vi "main.vi"() -> ()   [LabVIEW 2016]
uses:
  <vilib>/Utility/config.llb/Read Key (String).vi
  <vilib>/Utility/config.llb/Write Key (String).vi
  <vilib>/Utility/config.llb/NI_LVConfig.lvlib
  <vilib>/ptbypt/NI_PtbyPt.lvlib
panel:
  in  "Password":string="783523103"
  in  "日数据table表":string="t_sjzx_wryzxjc_fs_rsj"
  in  "connection information":string="mysql"
  out "计数":i32
  out "数值":i32
  out "time":string
  out "error out":errorcluster
  in  "修改数据发送起始时间":bool
  in  "因子编码表":bool
  in  "QYMC-企业名称":string="安徽晨蓝环保科技有限公司（凤台经济开发区污水处理厂）"
  in  "QYBH-企业编号":string="340100000133"
  in  "PKMC-排口名称":string="污水排口"
  in  "PKBH-排口编号":string="340400000010WaterOutput2"
  in  "XH-序号":string="34040000001020012018103012"
  in  "小时数据table表":string="t_sjzx_wryzxjc_fs_xssj"
  out "参数table":string
  out "数据时间":string[](array[string])
  in  "等待时间（毫秒）":u32=30000
  in  "参数数值":T1={"CODMn"=TRUE, "CODCr"=TRUE, "DO"=TRUE, "铜"=TRUE, "PH"=TRUE, "氨氮"=TRUE, "比电导率"=TRUE, "水温"=TRUE, "COD"=TRUE, "浊度"=TRUE, "总氮"=TRUE, "总磷"=TRUE, "叶绿素a"=TRUE, "藻密度"=TRUE, "水位"=TRUE, "流速"=TRUE, "瞬时流量"=TRUE, "累积流量"=TRUE, "亚硝氮"=TRUE, "硫化物"=TRUE, "ORP"=TRUE, "铅"=TRUE, "镉"=TRUE, "锌"=TRUE, "镍"=TRUE, "锰"=TRUE, "汞"=TRUE, "气温"=TRUE, "气压"=TRUE, "风速"=TRUE, "风向"=TRUE} caption="参数种类"
  # "定时分参数循环读取database数据------------->多条数据分条转换循环存储到mysql数据库中------->成功则更新搜索时间戳、失败不更新"
  # "示例：34040000001020012018103012"
  # "示例：340400000010WaterOutput2"
  # "示例：污水排口"
  # "示例：340100000133"
  # "示例：安徽晨蓝环保科技有限公司（凤台经济开发区污水处理厂）"
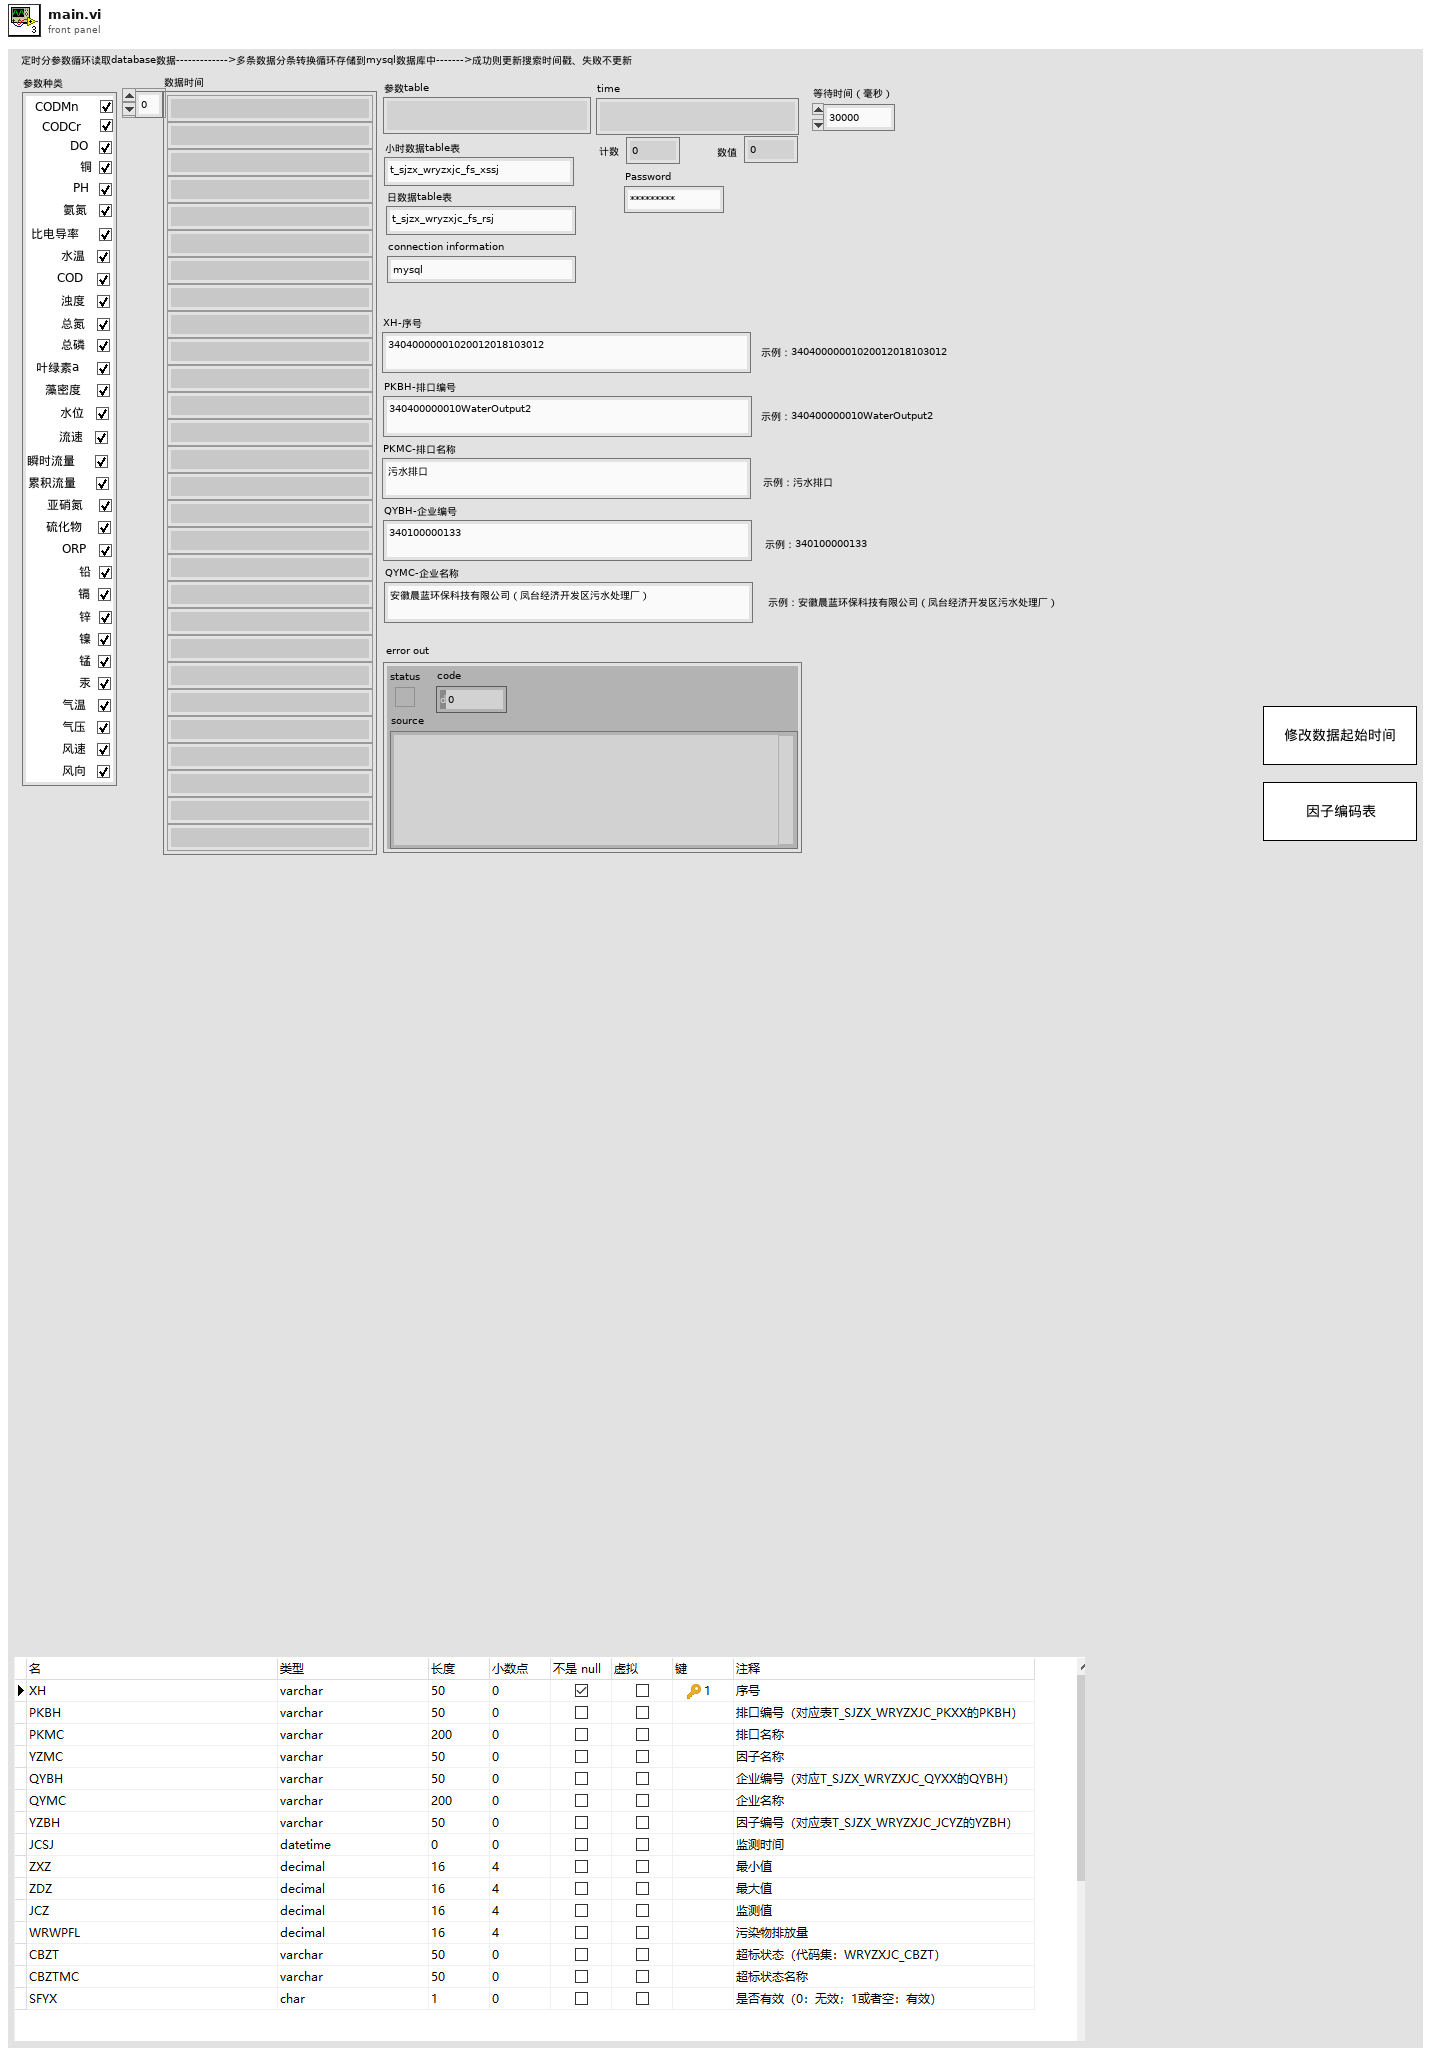
[diagram p1: front panel]
types:
  T1 = cluster{"CODMn":bool, "CODCr":bool, "DO":bool, "铜":bool, "PH":bool, "氨氮":bool, "比电导率":bool, "水温":bool, "COD":bool, "浊度":bool, "总氮":bool, "总磷":bool, "叶绿素a":bool, "藻密度":bool, "水位":bool, "流速":bool, "瞬时流量":bool, "累积流量":bool, "亚硝氮":bool, "硫化物":bool, "ORP":bool, "铅":bool, "镉":bool, "锌":bool, "镍":bool, "锰":bool, "汞":bool, "气温":bool, "气压":bool, "风速":bool, "风向":bool}
  T2 = typedef "NI_LVConfig.lvlib/Config Data RefNum.ctl" = refnum<k1>
  T3 = cluster{"[0]":string, "[1]":string, "[2]":string, "[3]":string, "[4]":string, "[5]":string, "[6]":string, "[7]":string, "[8]":string, "[9]":string, "[10]":string, "[11]":string, "[12]":string, "[13]":string, "[14]":string, "[15]":string, "[16]":string, "[17]":string, "[18]":string, "[19]":string, "[20]":string, "[21]":string, "[22]":string, "[23]":string, "[24]":string, "[25]":string, "[26]":string, "[27]":string, "[28]":string, "[29]":string, "[30]":string}
  T4 = typedef "LVDateTimeRec.ctl" = cluster{"秒数的小数部分":dbl, "秒":i32, "分":i32, "时":i32, "日":i32, "月":i32, "年":i32, "天数（周）":i32, "天数（年）":i32, "DST":i32}
  T5 = cluster{"CODMn":string, "CODCr":string, "DO":string, "铜":string, "PH":string, "氨氮":string, "比电导率":string, "水温":string, "COD":string, "浊度":string, "总氮":string, "总磷":string, "叶绿素a":string, "藻密度":string, "水位":string, "流速":string, "瞬时流量":string, "累积流量":string, "亚硝酸盐":string, "硫化物":string, "ORP":string, "铅":string, "镉":string, "锌":string, "镍":string, "锰":string, "汞":string, "气温":string, "气压":string, "风速":string, "风向":string}
  T6 = cluster{"XH":string, "PKBH":string, "PKMC":string, "YZBH":string, "YZMC":string, "QYBH":string, "QYMC":string, "JCSJ":timestamp, "JCZ":dbl}
  T7 = cluster{"time1":string, "time2":string, "time3":string, "time4":string, "time5":string, "time6":string, "time7":string, "time8":string, "time9":string, "time10":string, "time11":string, "time12":string, "time13":string, "time14":string, "time15":string, "time16":string, "time17":string, "time18":string, "time19":string, "time20":string, "time21":string, "time22":string, "time23":string, "time24":string, "time25":string, "time26":string, "time27":string, "time28":string, "time29":string, "time30":string, "time31":string}
  T8 = cluster{"XH":string, "PKBH":string, "PKMC":string, "YZMC":string, "QYBH":string, "QYMC":string, "YZBH":string, "JCSJ":timestamp, "JCZ":dbl}
  T9 = cluster{"配置表格[0]":string, "配置表格[1]":string, "配置表格[2]":string, "配置表格[3]":string, "配置表格[4]":string, "配置表格[5]":string, "配置表格[6]":string, "配置表格[7]":string, "配置表格[8]":string, "配置表格[9]":string, "配置表格[10]":string, "配置表格[11]":string, "配置表格[12]":string, "配置表格[13]":string, "配置表格[14]":string, "配置表格[15]":string, "配置表格[16]":string, "配置表格[17]":string, "配置表格[18]":string, "配置表格[19]":string, "配置表格[20]":string, "配置表格[21]":string, "配置表格[22]":string, "配置表格[23]":string, "配置表格[24]":string, "配置表格[25]":string, "配置表格[26]":string, "配置表格[27]":string, "配置表格[28]":string, "配置表格[29]":string, "配置表格[30]":string}
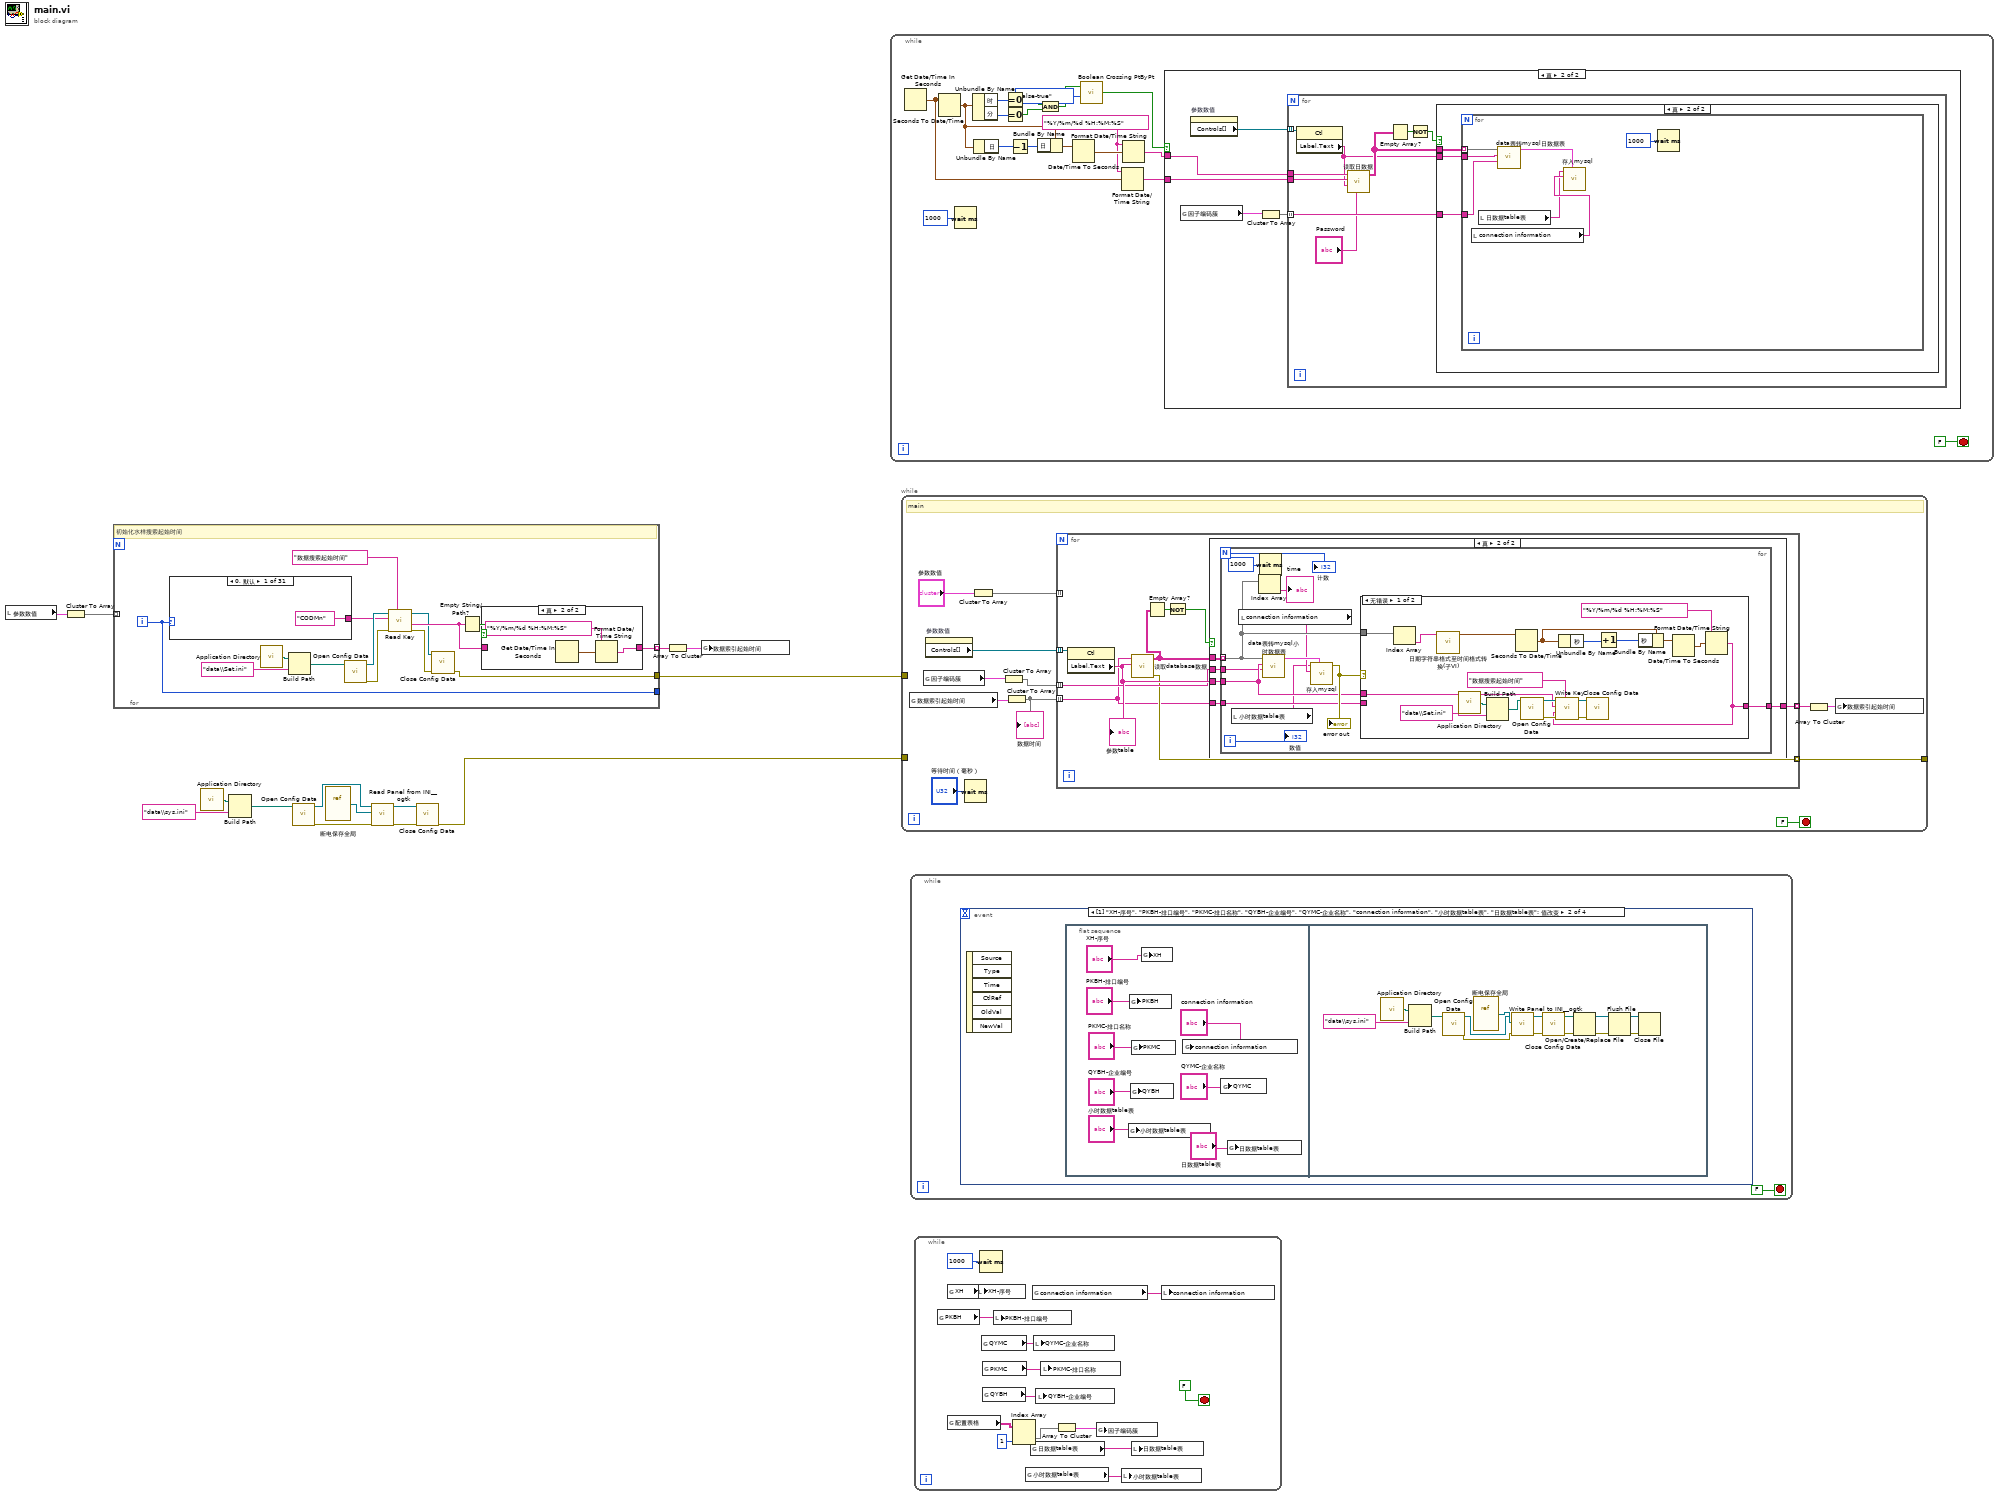
[diagram p0: block diagram]
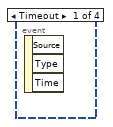
[diagram p4: hidden frame]
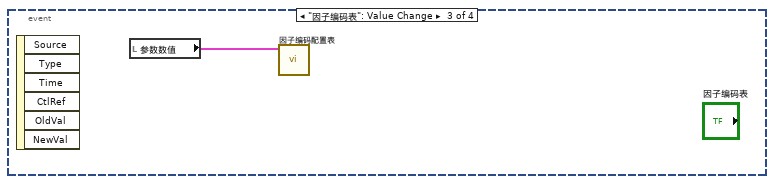
[diagram p5: hidden frame]
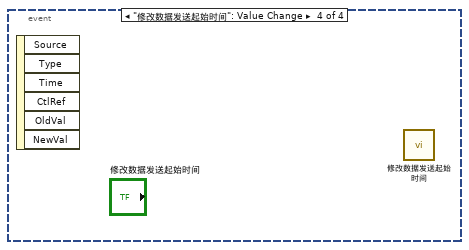
[diagram p6: hidden frame]
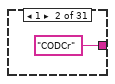
[diagram p8: hidden frame]
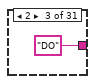
[diagram p9: hidden frame]
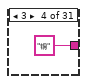
[diagram p10: hidden frame]
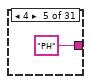
[diagram p11: hidden frame]
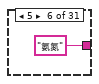
[diagram p12: hidden frame]
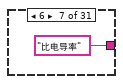
[diagram p13: hidden frame]
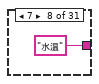
[diagram p14: hidden frame]
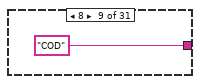
[diagram p15: hidden frame]
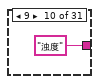
[diagram p16: hidden frame]
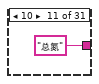
[diagram p17: hidden frame]
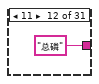
[diagram p18: hidden frame]
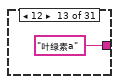
[diagram p19: hidden frame]
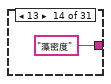
[diagram p20: hidden frame]
diagram:
  n1 = local read "参数数值"() -> (w14:T1)
  n2 = Cluster To Array(cluster=w14) -> (array=w13:bool[])
  n3 = for {
    tunnel: [w19] -> _
    tunnel: [w16] -> w12 mode=indexing
    tunnel: [w15] -> w11
    tunnel: w13 -> [_] mode=indexing
    i -> [w19]
    # "初始化水样搜索起始时间"
    n4 = case shown="0, 默认" w19 {
      tunnel: ["CODMn" "CODCr" "DO" "铜" "PH" "氨氮" "比电导率" "水温" "COD" "浊度" "总氮" "总磷" "叶绿素a" "藻密度" "水位" "流速" "瞬时流量" "累积流量" "亚硝氮" "硫化物" "ORP" "铅" "镉" "锌" "镍" "锰" "汞" "气温" "气压" "风速" "风向"] -> w22
      frame 0, Default {
      }
      frame 1 {
      }
      frame 2 {
      }
      frame 3 {
      }
      frame 4 {
      }
      frame 5 {
      }
      frame 6 {
      }
      frame 7 {
      }
      frame 8 {
      }
      frame 9 {
      }
      frame 10 {
      }
      frame 11 {
      }
      frame 12 {
      }
      frame 13 {
      }
      frame 14 {
      }
      frame 15 {
      }
      frame 16 {
      }
      frame 17 {
      }
      frame 18 {
      }
      frame 19 {
      }
      frame 20 {
      }
      frame 21 {
      }
      frame 22 {
      }
      frame 23 {
      }
      frame 24 {
      }
      frame 25 {
      }
      frame 26 {
      }
      frame 27 {
      }
      frame 28 {
      }
      frame 29 {
      }
      frame 30 {
      }
    }
    n5 = call <vilib>:"Application Directory.vi"() -> ("Application Directory"=w28:path)
    n6 = Build Path(base path=w28, name or relative path="data\\Set.ini" ("名称或相对路径")) -> (appended path=w26:path)
    n7 = call <vilib>:"Open Config Data.vi"("configuration file path"=w26) -> ("error out"=w24:errorcluster, "refnum"=w25:T2)  [unwired: 8 in, 1 out]
    n8 = call-poly <vilib>:"Read Key.vi"("section"="数据搜索起始时间", "error in (no error)"=w24, "key"=w22, "refnum"=w25) -> ("error out"=w17:errorcluster, "value"=w20:string, "refnum out"=w18:T2)  [unwired: 4 in, 1 out]
    n9 = call <vilib>:"Close Config Data.vi"("error in (no error)"=w17, "refnum"=w18) -> ("error out"=w15:errorcluster)  [unwired: 8 in, 1 out]
    n10 = Empty String/Path?(string/path=w20) -> (empty?=w21:bool)
    n11 = case shown="真" w21 {
      tunnel: [w29 w30] -> w16
      tunnel: w20 -> [w29 _]
      frame False {
      }
      frame True {
        n12 = Get Date/Time In Seconds() -> (seconds since 1Jan1904=w32:timestamp)
        n13 = Format Date/Time String(time format string (%c)="%Y/%m/%d %H:%M:%S" ("时间格式字符串(%c)"), seconds (now)=w32) -> (date/time string=w30:string)  [unwired: 1 in]
      }
    }
  }
  n14 = call <vilib>:"Application Directory.vi"() -> ("Application Directory"=w5:path)
  n15 = Build Path(base path=w5, name or relative path="data\\sys.ini" ("名称或相对路径")) -> (appended path=w3:path)
  n16 = call <vilib>:"Open Config Data.vi"("configuration file path"=w3) -> ("error out"=w9:errorcluster, "refnum"=w8:T2)  [unwired: 8 in, 1 out]
  n17 = vi-ref "断电保存全局.vi"() -> (w7:refnum<vi>)
  n18 = call <userlib>:"Read Panel from INI__ogtk.vi"("error in (no error)"=w9, "VI ref"=w7, "refnum"=w8) -> ("error out"=w2:errorcluster, "refnum out"=w6:T2)  [unwired: 7 in]
  n19 = call <vilib>:"Close Config Data.vi"("error in (no error)"=w2, "refnum"=w6) -> ("error out"=w1:errorcluster)  [unwired: 8 in, 1 out]
  n20 = Array To Cluster(array=w12) -> (cluster=w10:T3)
  n21 = global write "内部全局.vi" "数据索引起始时间"(w10) -> ()
  n22 = while {
    stop <- FALSE stop-if-true
    w70 = "%Y/%m/%d %H:%M:%S" ("时间格式字符串(%c)")
    n23 = Get Date/Time In Seconds() -> (seconds since 1Jan1904=w69:timestamp)
    n24 = Seconds To Date/Time(time stamp (now)=w69) -> (date time rec=w76:T4)  [unwired: 1 in]
    n25 = Wait (ms)(milliseconds to wait=u32 1000 ("等待时间（毫秒）")) -> ()  [unwired: 1 out]
    n26 = Unbundle By Name(w76) -> ("时"=w79:i32, "分"=w78:i32)
    n27 = Unbundle By Name(w76) -> ("日"=w75:i32)
    n28 = Equal To 0?(x=w79) -> (x = 0?=w72:bool)
    n29 = Equal To 0?(x=w78) -> (x = 0?=w73:bool)
    n30 = Decrement(x=w75) -> (x-1=w74:i32)
    n31 = Bundle By Name(cluster=w76, "日"=w74) -> (w77:T4)
    n32 = And(x=w72, y=w73) -> (x .and. y?=w66:bool)
    n33 = Date/Time To Seconds(2:w77) -> (0:w71:timestamp)  [unwired: 1 in]
    n34 = call <vilib>:"Boolean Crossing PtByPt.vi"("direction"=enum16{"either", "false-true", "true-false"}."false-true", "input"=w66) -> ("crossing"=w64:bool)  [unwired: 1 in]
    n35 = Format Date/Time String(time format string (%c)=w70, seconds (now)=w69) -> (date/time string=w67:string)  [unwired: 1 in]
    n36 = Format Date/Time String(time format string (%c)=w70, seconds (now)=w71) -> (date/time string=w68:string)  [unwired: 1 in]
    n37 = case shown="真" w64 {
      tunnel: w68 -> [_ w86]
      tunnel: w67 -> [_ w85]
      frame False {
      }
      frame True {
        n38 = global read "断电保存全局.vi" "因子编码簇"() -> (w83:T5)
        n39 = property on="参数数值" class="Clust (严格)"() -> ("Controls[]"=w84:refnum<vi>[])  [unwired: 2 in, 2 out]
        n40 = Cluster To Array(cluster=w83) -> (array=w82:string[])
        n41 = for {
          tunnel: w86 -> [w95]
          tunnel: w85 -> [w94]
          tunnel: w84 -> [w93] mode=indexing
          tunnel: w82 -> [w88] mode=indexing
          n42 = property class="Ctl"(reference=w93) -> ("Label.Text"=w89:string)  [unwired: 1 in, 2 out]
          n43 = call "读取日数据.vi"("Password"="Password", "table输入"=w89, "结束时间"=w94, "起始时间"=w95) -> ("data"=w90:string[][])  [unwired: 6 in, 1 out]
          n44 = Empty Array?(array=w90) -> (empty?=w92:bool)
          n45 = Not(x=w92) -> (.not. x?=w91:bool)
          n46 = case shown="真" w91 {
            tunnel: w90 -> [_ w98]
            tunnel: w89 -> [_ w97]
            tunnel: w88 -> [_ w96]
            frame False {
            }
            frame True {
              n47 = for {
                tunnel: w98 -> [w105] mode=indexing
                tunnel: w97 -> [w104]
                tunnel: w96 -> [w103]
                n48 = local read "connection information"() -> (w101:string)
                n49 = local read "日数据table表"() -> (w99:string)
                n50 = call "data表转mysql日数据表.vi"("YZBH"=w103, "YZMC"=w104, "data"=w105) -> ("mysqldata簇"=w102:T6)  [unwired: 8 in]
                n51 = call "存入mysql.vi"("mysqldata簇"=w102, "connection information"=w101, "table"=w99) -> ()  [unwired: 8 in, 1 out]
                n52 = Wait (ms)(milliseconds to wait=u32 1000 ("等待时间（毫秒）")) -> ()  [unwired: 1 out]
              }
            }
          }
        }
      }
    }
  }
  n53 = while {
    tunnel: w11 -> [_]
    tunnel: w1 -> [_]
    tunnel: [w108] -> _
    stop <- FALSE stop-if-true
    # "main"
    n54 = global read "内部全局.vi" "数据索引起始时间"() -> (w111:T7)
    n55 = global read "断电保存全局.vi" "因子编码簇"() -> (w110:T5)
    n56 = property on="参数数值" class="Clust (严格)"() -> ("Controls[]"=w113:refnum<vi>[])  [unwired: 2 in, 2 out]
    n57 = Wait (ms)(milliseconds to wait="等待时间（毫秒）") -> ()  [unwired: 1 out]
    n58 = Cluster To Array(cluster="参数数值") -> (array=w116:bool[])
    n59 = Cluster To Array(cluster=w110) -> (array=w109:string[])
    n60 = Cluster To Array(cluster=w111) -> (array=w112:string[])
    "数据时间" <- w112
    n61 = for {
      tunnel: w116 -> [_] mode=indexing
      tunnel: w113 -> [w126] mode=indexing
      tunnel: w112 -> [w122] mode=indexing
      tunnel: w109 -> [w124] mode=indexing
      tunnel: [w123] -> w108 mode=indexing
      tunnel: [w118] -> w107 mode=indexing
      n62 = property class="Ctl"(reference=w126) -> ("Label.Text"=w125:string)  [unwired: 1 in, 2 out]
      "参数table" <- w125
      n63 = call "读取database数据.vi"("table输入"=w125, "起始时间"=w122) -> ("error out"=w123:errorcluster, "data"=w120:string[][])  [unwired: 8 in]
      n64 = Empty Array?(array=w120) -> (empty?=w121:bool)
      n65 = Not(x=w121) -> (.not. x?=w119:bool)
      n66 = case shown="真" w119 {
        tunnel: w120 -> [_ w132]
        tunnel: w125 -> [_ w131]
        tunnel: w124 -> [_ w130]
        tunnel: w122 -> [w127 w129]
        tunnel: [w127 w128] -> w118
        frame False {
        }
        frame True {
          n67 = for {
            N -> [w137]
            tunnel: w132 -> [w141] mode=indexing
            tunnel: w131 -> [w144]
            tunnel: w130 -> [w142]
            tunnel: w129 -> [w135]
            tunnel: [w136] -> w128
            i -> [w138]
            n68 = local read "小时数据table表"() -> (w133:string)
            n69 = local read "connection information"() -> (w134:string)
            n70 = Index Array(array=w141) -> (element=→"time":string)  [unwired: 1 in]
            n71 = Wait (ms)(milliseconds to wait=u32 1000 ("等待时间（毫秒）")) -> ()  [unwired: 1 out]
            n72 = call "data表转mysql小时数据表.vi"("YZBH"=w142, "YZMC"=w144, "data"=w141) -> ("mysqldata簇"=w143:T8)  [unwired: 8 in]
            n73 = call "存入mysql.vi"("mysqldata簇"=w143, "connection information"=w134, "table"=w133) -> ("error out"=w145:errorcluster)  [unwired: 8 in]
            "error out" <- w145
            n74 = case shown="无错误" w145 {
              tunnel: w144 -> [w156 _]
              tunnel: w141 -> [w155 _]
              tunnel: [w146 w165] -> w136
              tunnel: w135 -> [_ w165]
              frame No Error {
                n75 = Index Array(array=w155) -> (element=w147:string)  [unwired: 1 in]
                n76 = call "日期字符串格式至时间格式转换(子VI).vi"("data[0]"=w147) -> ("time stamp"=w154:timestamp)  [unwired: 10 in]
                n77 = call <vilib>:"Application Directory.vi"() -> ("Application Directory"=w158:path)
                n78 = Build Path(base path=w158, name or relative path="data\\Set.ini" ("名称或相对路径")) -> (appended path=w160:path)
                n79 = Seconds To Date/Time(time stamp (now)=w154) -> (date time rec=w152:T4)  [unwired: 1 in]
                n80 = call <vilib>:"Open Config Data.vi"("configuration file path"=w160) -> ("error out"=w162:errorcluster, "refnum"=w161:T2)  [unwired: 8 in, 1 out]
                n81 = Unbundle By Name(w152) -> ("秒"=w153:i32)
                n82 = Increment(x=w153) -> (x+1=w151:i32)
                n83 = Bundle By Name(cluster=w152, "秒"=w151) -> (w149:T4)
                n84 = Date/Time To Seconds(2:w149) -> (0:w150:timestamp)  [unwired: 1 in]
                n85 = Format Date/Time String(time format string (%c)="%Y/%m/%d %H:%M:%S" ("时间格式字符串(%c)"), seconds (now)=w150) -> (date/time string=w146:string)  [unwired: 1 in]
                n86 = call-poly <vilib>:"Write Key.vi"("section"="数据搜索起始时间", "error in (no error)"=w162, "value"=w146, "key"=w156, "refnum"=w161) -> ("error out"=w164:errorcluster, "refnum out"=w163:T2)  [unwired: 4 in, 1 out]
                n87 = call <vilib>:"Close Config Data.vi"("error in (no error)"=w164, "refnum"=w163) -> ()  [unwired: 8 in, 2 out]
              }
              frame Error {
              }
            }
            "数值" <- w138
            "计数" <- w137
          }
        }
      }
    }
    n88 = Array To Cluster(array=w107) -> (cluster=w106:T3)
    n89 = global write "内部全局.vi" "数据索引起始时间"(w106) -> ()
  }
  n90 = while {
    stop <- FALSE stop-if-true
    n91 = event shown="[1] \"XH-序号\", \"PKBH-排口编号\", \"PKMC-排口名称\", \"QYBH-企业编号\", \"QYMC-企业名称\", \"connection information\", \"小时数据table表\", \"日数据table表\": 值改变" {
      selector: _ -> [_ _ _ _]
      dyn-events: _ -> [_ _ _ _]
      timeout: _ -> [_ _ _ _]
      event Timeout {
        n92 = event-data() -> ()  [unwired: 1 in, 3 out]
      }
      event "XH-序号", "PKBH-排口编号", "PKMC-排口名称", "QYBH-企业编号", "QYMC-企业名称", "connection information", "小时数据table表", "日数据table表": Value Change {
        n93 = event-data() -> ()  [unwired: 1 in, 6 out]
        n94 = flat-sequence {
          frame #0 {
            n95 = global write "断电保存全局.vi" "小时数据table表"("小时数据table表") -> ()
            n96 = global write "断电保存全局.vi" "PKBH"("PKBH-排口编号") -> ()
            n97 = global write "断电保存全局.vi" "QYBH"("QYBH-企业编号") -> ()
            n98 = global write "断电保存全局.vi" "PKMC"("PKMC-排口名称") -> ()
            n99 = global write "断电保存全局.vi" "XH"("XH-序号") -> ()
            n100 = global write "断电保存全局.vi" "connection information"("connection information") -> ()
            n101 = global write "断电保存全局.vi" "QYMC"("QYMC-企业名称") -> ()
            n102 = global write "断电保存全局.vi" "日数据table表"("日数据table表") -> ()
          }
          frame #1 {
            n103 = call <vilib>:"Application Directory.vi"() -> ("Application Directory"=w175:path)
            n104 = Build Path(base path=w175, name or relative path="data\\sys.ini" ("名称或相对路径")) -> (appended path=w177:path)
            n105 = call <vilib>:"Open Config Data.vi"("configuration file path"=w177) -> ("error out"=w181:errorcluster, "refnum"=w178:T2)  [unwired: 8 in, 1 out]
            n106 = vi-ref "断电保存全局.vi"() -> (w179:refnum<vi>)
            n107 = call <userlib>:"Write Panel to INI__ogtk.vi"("error in (no error)"=w181, "VI ref"=w179, "refnum"=w178) -> ("error out"=w182:errorcluster, "refnum out"=w180:T2)  [unwired: 7 in]
            n108 = call <vilib>:"Close Config Data.vi"("error in (no error)"=w182, "refnum"=w180) -> ("error out"=w187:errorcluster, "file path"=w188:path)  [unwired: 8 in]
            n109 = Open/Create/Replace File(file path (use dialog)=w188, error in=w187) -> (refnum out=w184:refnum<file>, error out=w183:errorcluster)  [unwired: 4 in, 1 out]
            n110 = Flush File(refnum=w184, error in=w183) -> (refnum out=w185:refnum<file>, error out=w186:errorcluster)
            n111 = Close File(refnum=w185, error in=w186) -> ()  [unwired: 2 out]
          }
        }
      }
      event "因子编码表": Value Change {
        n112 = event-data() -> ()  [unwired: 1 in, 6 out]
        n113 = local read "参数数值"() -> (w189:T1)
        n114 = call "因子编码配置表.vi"("参数数值"=w189) -> ()  [unwired: 11 in]
      }
      event "修改数据发送起始时间": Value Change {
        n115 = event-data() -> ()  [unwired: 1 in, 6 out]
        n116 = call "修改数据发送起始时间.vi"() -> ()  [unwired: 12 in]
      }
    }
  }
  n117 = while {
    stop <- FALSE stop-if-true
    n118 = global read "断电保存全局.vi" "PKBH"() -> (w200:string)
    n119 = global read "断电保存全局.vi" "XH"() -> (w201:string)
    n120 = global read "断电保存全局.vi" "配置表格"() -> (w196:string[][])
    n121 = local write "XH-序号"(w201) -> ()
    n122 = Wait (ms)(milliseconds to wait=u32 1000 ("等待时间（毫秒）")) -> ()  [unwired: 1 out]
    n123 = global read "断电保存全局.vi" "QYMC"() -> (w197:string)
    n124 = global read "断电保存全局.vi" "PKMC"() -> (w199:string)
    n125 = global read "断电保存全局.vi" "QYBH"() -> (w198:string)
    n126 = local write "PKBH-排口编号"(w200) -> ()
    n127 = Index Array(array=w196, index (col)=1 ("禁用的索引 (列)")) -> (element=w194:string[])  [unwired: 1 in]
    n128 = global read "断电保存全局.vi" "小时数据table表"() -> (w191:string)
    n129 = global read "断电保存全局.vi" "日数据table表"() -> (w190:string)
    n130 = global read "断电保存全局.vi" "connection information"() -> (w192:string)
    n131 = local write "QYMC-企业名称"(w197) -> ()
    n132 = local write "QYBH-企业编号"(w198) -> ()
    n133 = local write "PKMC-排口名称"(w199) -> ()
    n134 = Array To Cluster(array=w194) -> (cluster=w193:T9)
    n135 = global write "断电保存全局.vi" "因子编码簇"(w193) -> ()
    n136 = local write "小时数据table表"(w191) -> ()
    n137 = local write "日数据table表"(w190) -> ()
    n138 = local write "connection information"(w192) -> ()
  }
